vi "clear caution status flag.vi"(8 "error in (no error)":errorcluster) -> (0 "error out":errorcluster)   [LabVIEW 2024, in "atsj peakcan basic.lvlib"]
doc: "Clears the <b>caution</b> flag from the error cluster.\n\nCopyright (c) 2025 ATSJ (www.atsj.eu)"
uses:
  atsj peakcan basic.lvlib
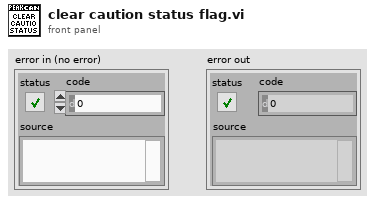
[diagram p1: front panel]
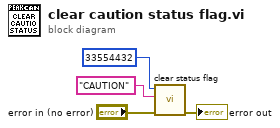
[diagram p0: block diagram]
diagram:
  n1 = call "clear status flag.vi"("error in (no error)"="error in (no error)", "flag name to clear"="CAUTION", "flag to clear"=u32 33554432) -> ("error out"=→"error out":errorcluster)  [unwired: 8 in]
